vi "Read KIT Calibration Files.vi"(8 "Error In":errorcluster, 11 "KIT-QA in":refnum<class "KIT-QA.lvclass">) -> (0 "Error Out":errorcluster, 3 "KIT-QA out":refnum<class "KIT-QA.lvclass">)   [LabVIEW 2015, in "KIT-QA.lvlib" / "KIT-QA.lvclass"]
doc: "Read calibration files to be used from separate configuration."
uses:
  KIT-QA.lvclass
  KIT-QA.lvclass/KIT-QA.ctl
  CSPP_Core/Actors/CS++BaseActor/CS++BaseActor.lvclass/CS++BaseActor.ctl
  <vilib>/Utility/config.llb/Read Key (String).vi
  <vilib>/Utility/config.llb/Read Key (Double).vi
  CSPP_Core/Actors/CS++BaseActor/CS++BaseActor.lvclass
  <vilib>/Utility/config.llb/NI_LVConfig.lvlib
  CSPP_Core/Libraries/Utilities/CS++Utilities.lvlib
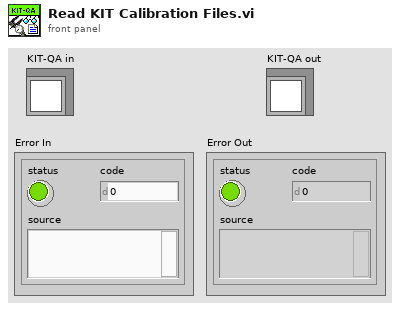
[diagram p1: front panel]
types:
  T1 = typedef "NI_LVConfig.lvlib/Config Data RefNum.ctl" = refnum<k1>
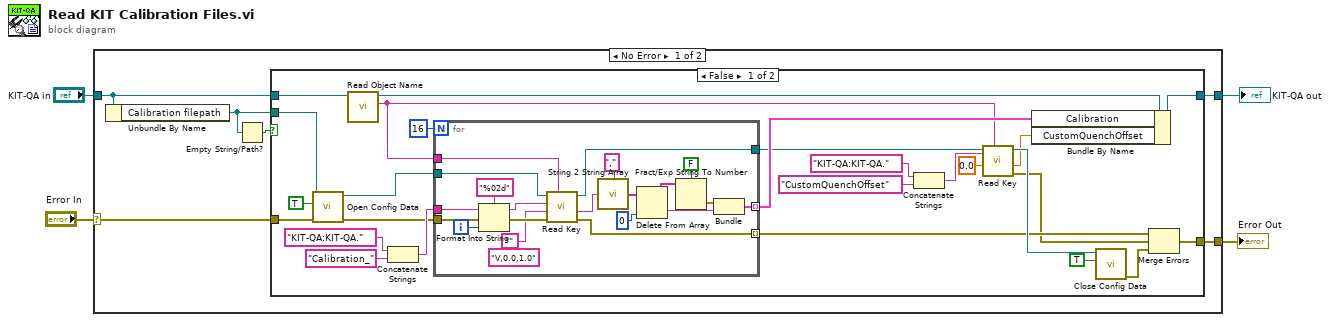
[diagram p0: block diagram]
diagram:
  n1 = case shown="No Error" "Error In" {
    selector: "Error In" -> [w10 w60]
    tunnel: [w7 w60] -> w3
    tunnel: [w8 w59] -> w1
    tunnel: "KIT-QA in" -> [w9 w59]
    frame No Error {
      n2 = Unbundle By Name(w9) -> ("Calibration filepath"=w6:path)
      n3 = Empty String/Path?(string/path=w6) -> (empty?=w5:bool)
      n4 = case shown="False" w5 {
        tunnel: w6 -> [w29 _]
        tunnel: w10 -> [w27 w57]
        tunnel: w9 -> [w36 w58]
        tunnel: [w31 w58] -> w8
        tunnel: [w30 w57] -> w7
        frame False {
          n5 = call <vilib>:"Open Config Data.vi"("error in (no error)"=w27, "create file if necessary (T)"=TRUE, "configuration file path"=w29) -> ("error out"=w24:errorcluster, "refnum"=w26:T1)  [unwired: 6 in, 1 out]
          n6 = call "Read Object Name.vi"("CS++BaseActor in"=w36) -> ("Object Name"=w11:string, "CS++BaseActor out"=w32:refnum<class "KIT-QA.lvclass">)  [unwired: 8 in, 1 out]
          n7 = Concatenate Strings("KIT-QA:KIT-QA.", "Calibration_" ("string")) -> (w33:string)
          n8 = for {
            N: 16 -> [_]
            tunnel: w33 -> [w56]
            tunnel: w26 -> [w53]
            tunnel: w24 -> [w52]
            tunnel: [w38] -> w16 mode=indexing
            tunnel: w11 -> [w50]
            tunnel: [w49] -> w17
            tunnel: [w39] -> w22 mode=indexing
            i -> [w55]
            (unwired) "V,0.0,1.0" ("String")
            n9 = Format Into String(format string="%02d", initial string=w56, error in=w52, w55) -> (resulting string=w54:string, error out=w51:errorcluster)
            n10 = call-poly <vilib>:"Read Key.vi"("section"=w50, "error in (no error)"=w51, "default value"="", "key"=w54, "refnum"=w53) -> ("error out"=w38:errorcluster, "value"=w40:string, "refnum out"=w49:T1)  [unwired: 3 in, 1 out]
            n11 = call "String 2 String Array.vi"("String"=w40, "Delimiter (\",\")"="," ("Delimiter (\",\")")) -> ("Substrings"=w46:string[])
            n12 = Delete From Array(array=w46, index=0) -> (deleted portion=w42:string, array with subset deleted=w43:string[])  [unwired: 1 in]
            n13 = Fract/Exp String To Number(use system decimal point (T)=FALSE, string=w43) -> (number=w44:dbl[])  [unwired: 2 in, 1 out]
            n14 = Bundle(w44, "Substring"=w42) -> (w39:cluster{dbl[], "Substring":string})  [unwired: 1 in]
          }
          n15 = Concatenate Strings("KIT-QA:KIT-QA.", "CustomQuenchOffset" ("string")) -> (w19:string)
          n16 = call-poly <vilib>:"Read Key.vi"("section"=w11, "default value"=0.0, "key"=w19, "refnum"=w17) -> ("error out"=w14:errorcluster, "value"=w13:dbl, "refnum out"=w18:T1)  [unwired: 4 in, 1 out]
          n17 = Bundle By Name(cluster=w32, "Calibration"=w22, "CustomQuenchOffset"=w13) -> (w31:refnum<class "KIT-QA.lvclass">)
          n18 = call <vilib>:"Close Config Data.vi"("write file if changed (T)"=TRUE, "refnum"=w18) -> ("error out"=w15:errorcluster)  [unwired: 8 in, 1 out]
          n19 = Merge Errors(w16, w14, w15) -> (w30:errorcluster)
        }
        frame True {
        }
      }
    }
    frame Error {
    }
  }
  "Error Out" <- w3
  "KIT-QA out" <- w1
